vi "eyeblink conditioning system.vi"() -> ()   [LabVIEW 2014]
panel:
  in  "change settings dir":bool
  in  "exit":bool
  in  "analyze data":bool
  in  "acquire data":bool
  # "animal version June 2010"
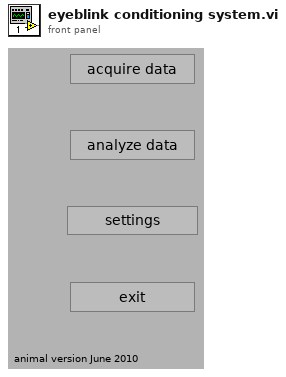
[diagram p1: front panel]
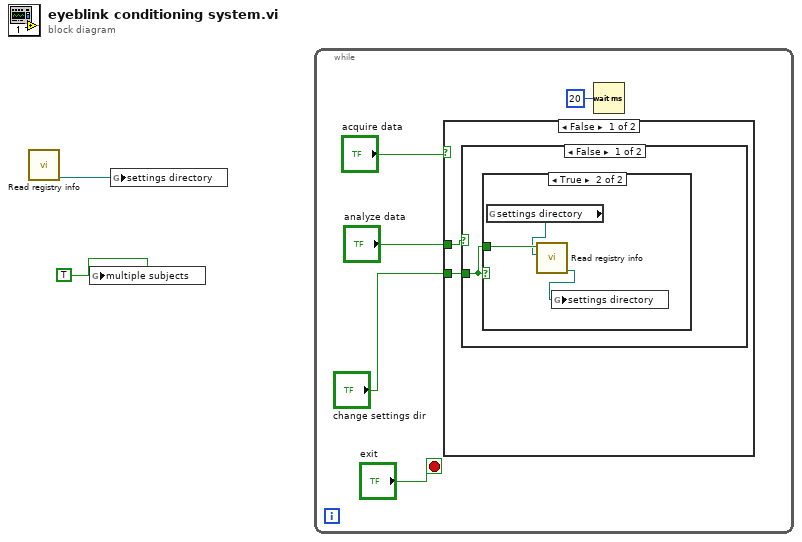
[diagram p0: block diagram]
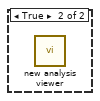
[diagram p3: hidden frame]
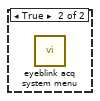
[diagram p4: hidden frame]
diagram:
  n1 = call "Read registry info.vi"() -> ("settings directory"=w2:path)  [unwired: 11 in]
  n2 = global write "acquisition globals" "multiple subjects"(TRUE ("multiple subjects")) -> ()
  n3 = global write "global settings" "settings directory"(w2) -> ()
  n4 = while {
    stop <- "exit" stop-if-true
    n5 = case shown="False" "acquire data" {
      tunnel: "analyze data" -> [w9 _]
      tunnel: "change settings dir" -> [w8 _]
      frame False {
        n6 = case shown="False" w9 {
          tunnel: w8 -> [w10 _]
          frame False {
            n7 = case shown="True" w10 {
              tunnel: w10 -> [_ w13]
              frame False {
              }
              frame True {
                n8 = global read "global settings" "settings directory"() -> (w12:path)
                n9 = call "Read registry info.vi"("settings directory in"=w12, "change directory"=w13) -> ("settings directory"=w11:path)  [unwired: 9 in]
                n10 = global write "global settings" "settings directory"(w11) -> ()
              }
            }
          }
          frame True {
            n11 = call "new analysis viewer.vi"() -> ()  [unwired: 8 in]
          }
        }
      }
      frame True {
        n12 = call "eyeblink acq system menu"() -> ()  [unwired: 1 in]
      }
    }
    n13 = Wait (ms)(milliseconds to wait=u32 20) -> ()  [unwired: 1 out]
  }
